vi "Linear Pixel to Angle Aproximation.vi"(1 "Axis Pixel":dbl, 2 "Axis Fov":dbl, 3 "Axis Lengh":dbl) -> (0 "Angle":dbl)   [LabVIEW 2016]
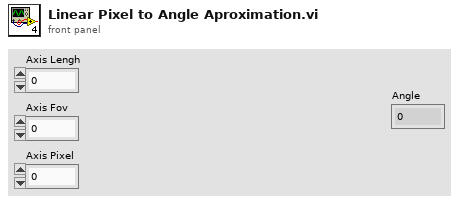
[diagram p1: front panel]
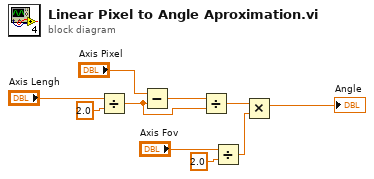
[diagram p0: block diagram]
diagram:
  n1 = Divide(x="Axis Lengh", y=2.0) -> (x/y=w2:dbl)
  n2 = Subtract(x="Axis Pixel", y=w2) -> (x-y=w7:dbl)
  n3 = Divide(x=w7, y=w2) -> (x/y=w3:dbl)
  n4 = Divide(x="Axis Fov", y=2.0) -> (x/y=w4:dbl)
  n5 = Multiply(x=w3, y=w4) -> (x*y=→"Angle":dbl)
